vi "Read FFID_Header.vi"(0 "Raw Data header String":string) -> (1 "Ch names":string[](array[string]), 2 "FFID Header Info":string[][](array[string]), 3 "Bkgnd Volts Present?":bool)   [LabVIEW 2022 SP3]
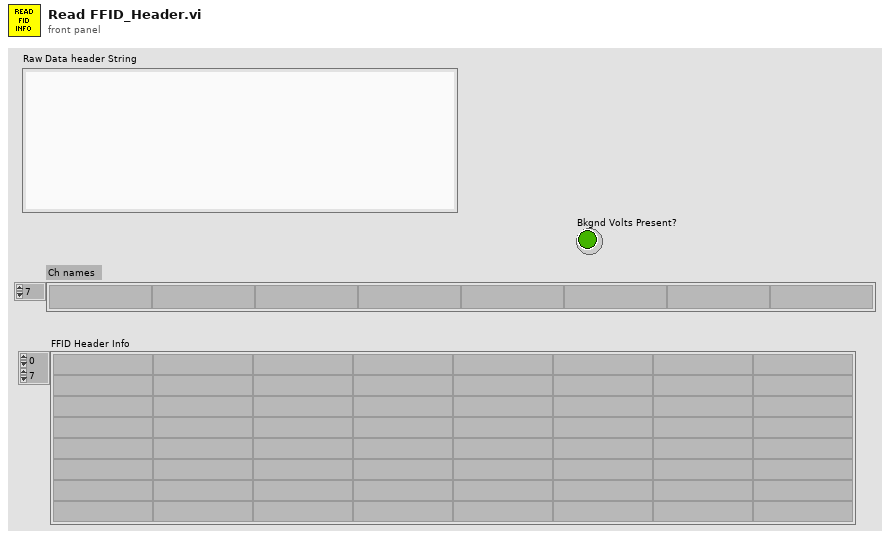
[diagram p1: front panel]
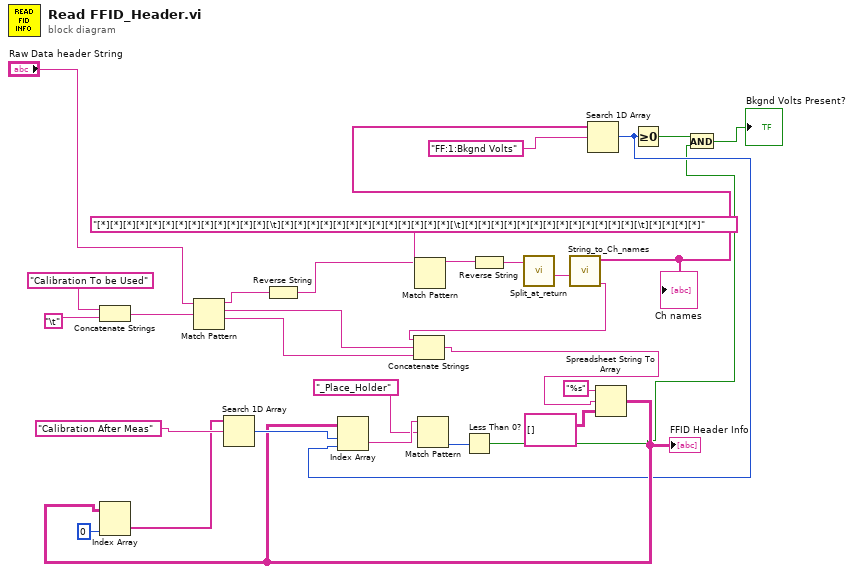
[diagram p0: block diagram]
diagram:
  n1 = Concatenate Strings("Calibration To be Used" ("Input Element"), "\t") -> (w17:string)
  n2 = Match Pattern(string="Raw Data header String", regular expression=w17) -> (before substring=w22:string, match substring=w28:string, after substring=w29:string)  [unwired: 2 out]
  n3 = Reverse String(1:w22) -> (0:w23:string)
  n4 = Match Pattern(string=w23, regular expression="[*][*][*][*][*][*][*][*][*][*][*][*][*][\t][*][*][*][*][*][*][*][*][*][*][*][*][*][\t][*][*][*][*][*][*][*][*][*][*][*][*][*][\t][*][*][*][*]" ("String")) -> (before substring=w21:string)  [unwired: 4 out]
  n5 = Reverse String(1:w21) -> (0:w20:string)
  n6 = call "Split_at_return.vi"("String"=w20) -> ("after substring"=w19:string)  [unwired: 1 in, 3 out]
  n7 = call "String_to_Ch_names.vi"("Spreadsheet string"=w19) -> ("Ch names"=w14:string[], "String After names"=w27:string)  [unwired: 2 out]
  "Ch names" <- w14
  n8 = Concatenate Strings(w27, w28, w29) -> (w30:string)
  n9 = Search 1D Array(1D array=w14, element="FF:1:Bkgnd Volts") -> (index of element=w8:i32)  [unwired: 1 out]
  n10 = Spreadsheet String To Array(format string="%s", spreadsheet string=w30, array type (2D Dbl)=string[][] []) -> (array=w9:string[][])  [unwired: 1 out]
  "FFID Header Info" <- w9
  n11 = Index Array(array=w9, index (col)=0 ("disabled index (col)")) -> (element=w11:string[])  [unwired: 1 in]
  n12 = Search 1D Array(1D array=w11, element="Calibration After Meas") -> (index of element=w10:i32)  [unwired: 1 out]
  n13 = Index Array(array=w9, index (row)=w10, index (col)=w8) -> (element=w7:string)
  n14 = Match Pattern(string=w7, regular expression="_Place_Holder") -> (offset past match=w5:i32)  [unwired: 4 out]
  n15 = Less Than 0?(x=w5) -> (x < 0?=w3:bool)
  n16 = Greater Or Equal To 0?(x=w8) -> (x >= 0?=w4:bool)
  n17 = And(x=w4, y=w3) -> (x .and. y?=→"Bkgnd Volts Present?":bool)
